vi "test_all.vi"() -> (3 "all_passed":bool)   [LabVIEW 2019]
doc: "Tests all Hashlib VIs"
panel:
  out "passed":bool[](array[boolean])
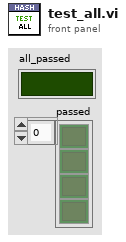
[diagram p1: front panel]
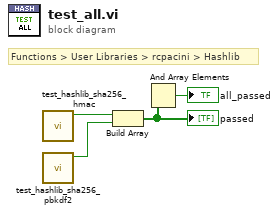
[diagram p0: block diagram]
diagram:
  # "Functions > User Libraries > rcpacini > Hashlib"
  n1 = call "test_hashlib_sha256_hmac.vi"() -> ("all_passed"=w3:bool)  [unwired: 11 in]
  n2 = call "test_hashlib_sha256_pbkdf2.vi"() -> ("all_passed"=w2:bool)  [unwired: 11 in]
  n3 = Build Array(w3, w2) -> (w1:bool[])
  "passed" <- w1
  n4 = And Array Elements(Boolean array=w1) -> (logical AND=→"all_passed":bool)
